vi "Update display target.vi"(8 "error in (no error)":errorcluster, 11 "StageSPIM in":refnum<class "StageSPIM.lvclass">) -> (0 "error out":errorcluster, 3 "StageSPIM out":refnum<class "StageSPIM.lvclass">)   [LabVIEW 2012, in "StageSPIM.lvclass"]
uses:
  StageSPIM.lvclass
  StageSPIM.lvclass/StageSPIM.ctl
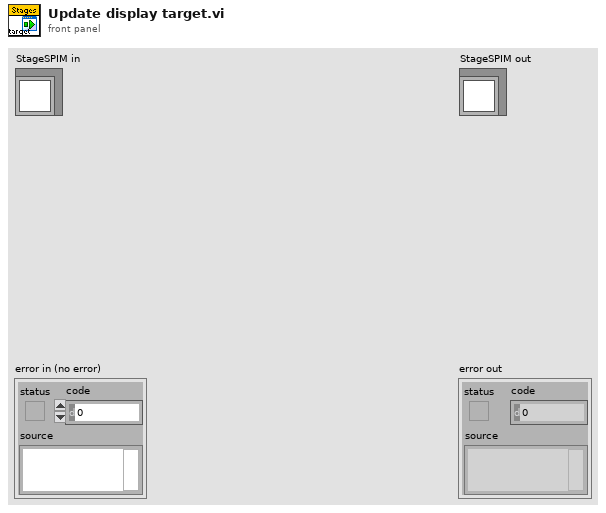
[diagram p1: front panel]
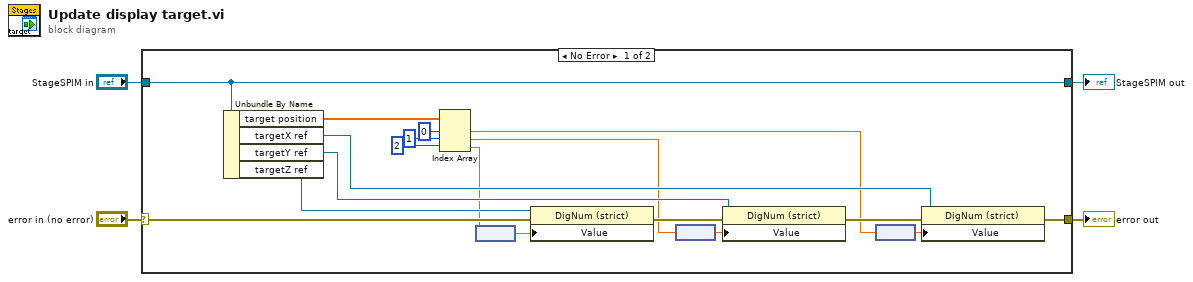
[diagram p0: block diagram]
diagram:
  n1 = case shown="No Error" "error in (no error)" {
    selector: "error in (no error)" -> [w9 w24]
    tunnel: [w8 w24] -> w3
    tunnel: [w10 w23] -> w1
    tunnel: "StageSPIM in" -> [w10 w23]
    frame No Error {
      n2 = Unbundle By Name(w10) -> ("target position"=w22:dbl[], "targetX ref"=w16:refnum<vi>, "targetY ref"=w17:refnum<vi>, "targetZ ref"=w18:refnum<vi>)
      n3 = Index Array(array=w22, index #1=0 ("index"), index #2=1 ("index"), index #3=2 ("index")) -> (element #1=w7:dbl, element #2=w6:dbl, element #3=w5:dbl)
      n4 = node(w5) -> (w13:dbl[unit])
      n5 = property class="DigNum (strict)"(reference=w18, error in=w9, "Value"=w13) -> (error out=w15:errorcluster)  [unwired: 1 out]
      n6 = node(w6) -> (w12:dbl[unit])
      n7 = property class="DigNum (strict)"(reference=w17, error in=w15, "Value"=w12) -> (error out=w14:errorcluster)  [unwired: 1 out]
      n8 = node(w7) -> (w11:dbl[unit])
      n9 = property class="DigNum (strict)"(reference=w16, error in=w14, "Value"=w11) -> (error out=w8:errorcluster)  [unwired: 1 out]
    }
    frame Error {
    }
  }
  "error out" <- w3
  "StageSPIM out" <- w1
